vi "dfd_h(n) Scaling.vi"(7 "L":i32, 9 "scale type":T1=enum."Time Domain 1-Norm", 10 "scale by Power of 2?":bool, 11 "h(n)":dbl[](array[numeric])) -> (1 "norm value":dbl, 2 "scale value":dbl, 3 "scaled  h(n)":dbl[](array[numeric]))   [LabVIEW 2017, in "NI_DigFilter_FXP.lvlib"]
uses:
  <vilib>/addons/Digital Filter Design/NI_DigFilter_FXP.lvlib
  <vilib>/addons/Digital Filter Design/_Objects.llb/DFD Coef Norm Type.ctl
  <vilib>/addons/Digital Filter Design/NI_DigFilterLicensed.lvlib
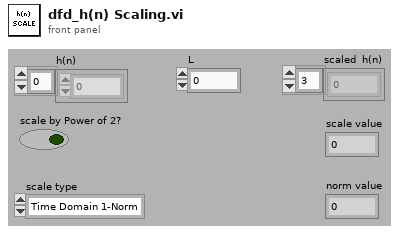
[diagram p1: front panel]
types:
  T1 = typedef "NI_DigFilterLicensed.lvlib/DFD Coef Norm Type.ctl" = enum16{"No Norm", "Time Domain 1-Norm", "Time Domain 2-Norm", "Time Domain Inf-Norm"}
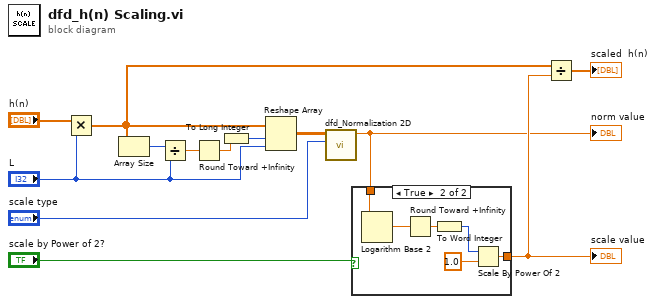
[diagram p0: block diagram]
diagram:
  n1 = Multiply(x="h(n)", y="L") -> (x*y=w2:dbl[])
  n2 = Array Size(array=w2) -> (size(s)=w10:i32)
  n3 = Divide(x=w10, y="L") -> (x/y=w9:dbl)
  n4 = Round Toward +Infinity(x=w9) -> (ceil(x): smallest int >= x=w8:dbl)
  n5 = To Long Integer(number=w8) -> (32bit integer=w7:i32)
  n6 = Reshape Array(w2, w7, "L") -> (w6:dbl[][])
  n7 = call <vilib>:"dfd_Normalization 2D.vi"("scale type"="scale type", "2D Array (col-major)"=w6) -> ("max norm"=w4:dbl)  [unwired: 9 out]
  "norm value" <- w4
  n8 = case shown="True" "scale by Power of 2?" {
    tunnel: w4 -> [w14 w18]
    tunnel: [w14 w15] -> w11
    frame False {
    }
    frame True {
      n9 = Logarithm Base 2(1:w18) -> (0:w20:dbl)
      n10 = Round Toward +Infinity(x=w20) -> (ceil(x): smallest int >= x=w19:dbl)
      n11 = To Word Integer(number=w19) -> (16bit integer=w16:i16)
      n12 = Scale By Power Of 2(n=w16, x=1.0) -> (x*2^n=w15:dbl)
    }
  }
  "scale value" <- w11
  n13 = Divide(x=w2, y=w11) -> (x/y=→"scaled  h(n)":dbl[])
